vi "Add Waveform.vi"(8 "error in (no error)":errorcluster, 10 "Waveform.lvclass":refnum<class "Waveform.lvclass">, 11 "Composite Waveform in":refnum<class "Composite Waveform.lvclass">) -> (0 "error out":errorcluster, 3 "Composite Waveform out":refnum<class "Composite Waveform.lvclass">)   [LabVIEW 2016, in "Composite Waveform.lvclass"]
uses:
  Composite Waveform.lvclass
  Waveform/Waveform.lvclass
  Composite Waveform.lvclass/Composite Waveform.ctl
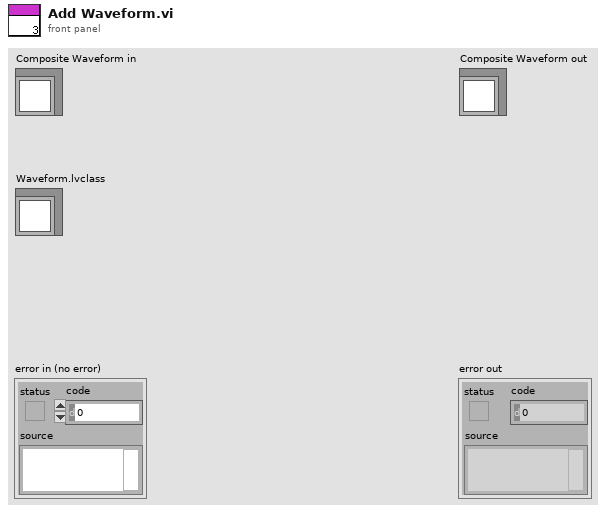
[diagram p1: front panel]
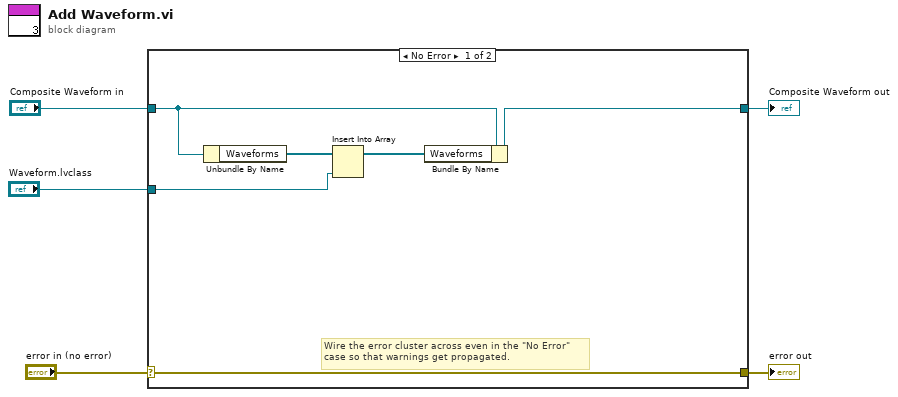
[diagram p0: block diagram]
diagram:
  n1 = case shown="No Error" "error in (no error)" {
    selector: "error in (no error)" -> [w11 w13]
    tunnel: [w11 w13] -> w4
    tunnel: [w8 w12] -> w2
    tunnel: "Composite Waveform in" -> [w10 w12]
    tunnel: "Waveform.lvclass" -> [w6 _]
    frame No Error {
      # "Wire the error cluster across even in the \"No Error\"\ncase so that warnings get propagated."
      n2 = Unbundle By Name(w10) -> ("Waveforms"=w9:refnum<class "Waveform.lvclass">[])
      n3 = Insert Into Array(array=w9, new element=w6) -> (w7:refnum<class "Waveform.lvclass">[])  [unwired: 1 in]
      n4 = Bundle By Name(cluster=w10, "Waveforms"=w7) -> (w8:refnum<class "Composite Waveform.lvclass">)
    }
    frame Error {
    }
  }
  "error out" <- w4
  "Composite Waveform out" <- w2
